vi "One Tolerant Inputs.vi"(8 "error in (no error)":errorcluster, 10 "Tolerance":dbl, 11 "Mock in":refnum<class "LMock Mock.lvclass">) -> (0 "error out":errorcluster, 3 "Mock out":refnum<class "LMock Mock.lvclass">)   [LabVIEW 2020, in "One.lvlib"]
uses:
  One.lvlib
  Framework/Mock/LMock Mock.lvclass
  Comparators/Tolerant Numeric Input Comparator/Tolerant Numeric Input Comparator.lvclass/Tolerant Numeric Input Comparator.ctl
  Comparators/Tolerant Numeric Input Comparator/Tolerant Numeric Input Comparator.lvclass
  C:/git/astemes-lmock/source/Core/Comparator/Comparator.lvclass
  One.lvclass
  C:/git/astemes-lmock/source/Core/Expectation/Expectation.lvclass
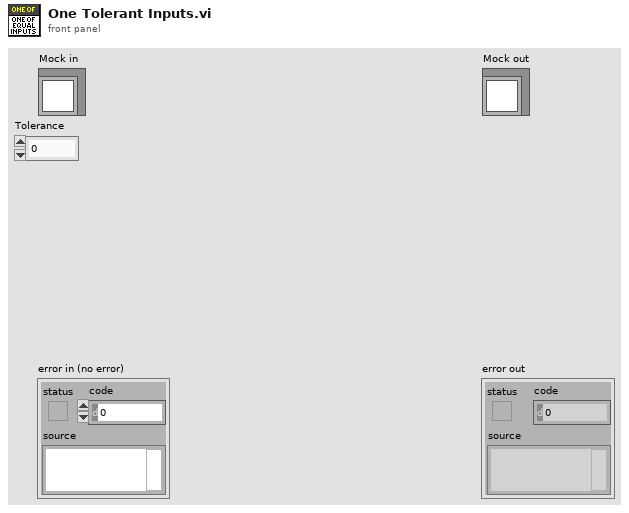
[diagram p1: front panel]
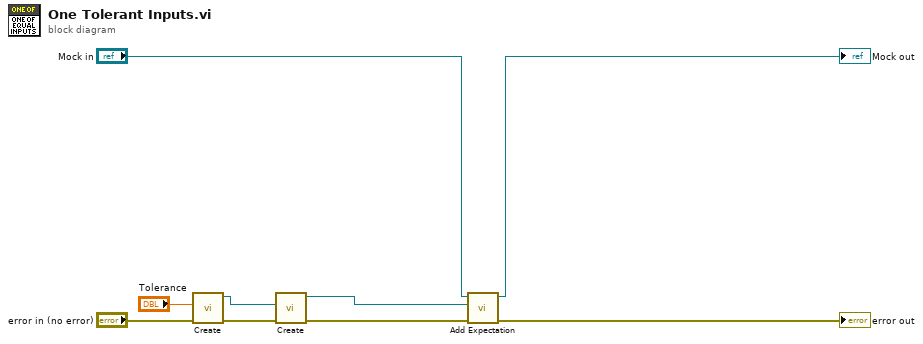
[diagram p0: block diagram]
diagram:
  n1 = call "Create.vi"("error in (no error)"="error in (no error)", "Tolerance"="Tolerance") -> ("error out"=w2:errorcluster, "Tolerant Numeric Comparator Out"=w4:refnum<class "Tolerant Numeric Input Comparator.lvclass">)  [unwired: 8 in]
  n2 = call "Create.vi"("error in (no error)"=w2, "Comparator"=w4) -> ("error out"=w6:errorcluster, "One"=w5:refnum<class "One.lvclass">)  [unwired: 8 in]
  n3 = call-dynamic "Add Expectation.vi"("error in (no error)"=w6, "Expectations"=w5, "Mock in"="Mock in") -> ("error out"=→"error out":errorcluster, "Mock out"=→"Mock out":refnum<class "LMock Mock.lvclass">)  [unwired: 7 in]
